vi "GetAppRefnum.vi"(8 "error in (no error)":errorcluster, 11 "CodeCoverage in":refnum<class "CodeCoverage.lvclass">) -> (0 "error out":errorcluster, 2 "App Refnum":refnum<vi>, 3 "CodeCoverage out":refnum<class "CodeCoverage.lvclass">)   [LabVIEW 2017, in "CodeCoverage.lvclass"]
doc: "Returns the application refnum for the context monitored by the code coverage module."
uses:
  CodeCoverage.lvclass
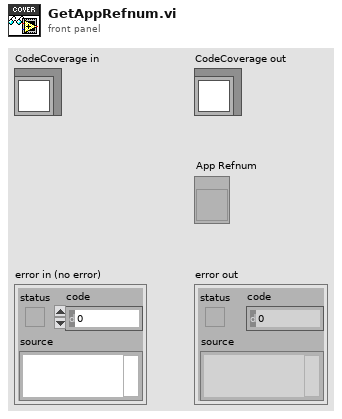
[diagram p1: front panel]
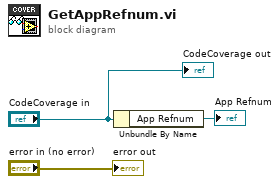
[diagram p0: block diagram]
diagram:
  n1 = Unbundle By Name("CodeCoverage in") -> ("App Refnum"=→"App Refnum":refnum<vi>)
  "error out" <- "error in (no error)"
  "CodeCoverage out" <- "CodeCoverage in"
